vi "Unregister User Event.vi"(8 "error in (no error)":errorcluster, 10 "Event Registration in":refnum<event-registration>, 11 "Session in":refnum<k21>) -> (0 "error out":errorcluster, 3 "Session out":refnum<k21>)   [LabVIEW 2020, in "nisyscfg.lvlib"]
uses:
  <vilib>/nisyscfg/nisyscfg.lvlib
  <vilib>/nisyscfg/User Event.ctl
panel:
  in  "System Configuration":refnum<user-event>
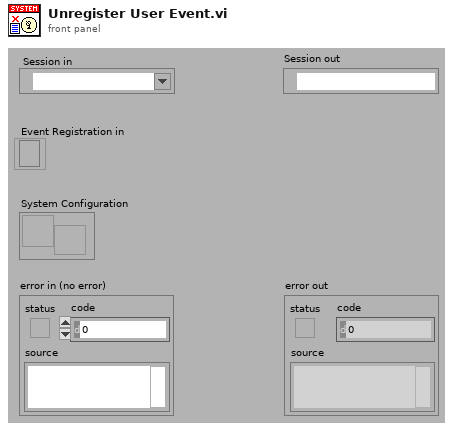
[diagram p1: front panel]
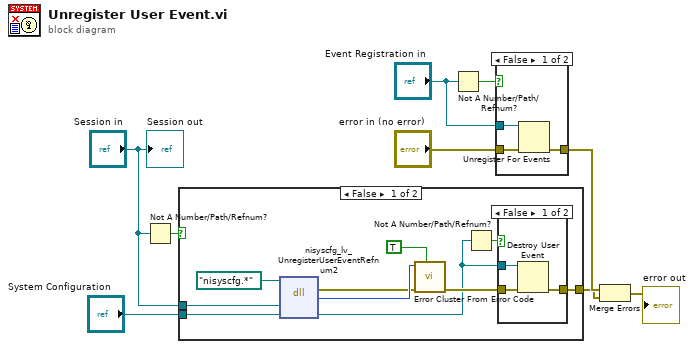
[diagram p0: block diagram]
diagram:
  n1 = Not A Number/Path/Refnum?(number/path/refnum="Session in") -> (NaN/Path/Refnum?=w5:bool)
  n2 = case shown="False" w5 {
    tunnel: [w13 _] -> w2
    tunnel: "Session in" -> [w17 _]
    tunnel: "System Configuration" -> [w12 _]
    frame False {
      n3 = dll-call lib="nisyscfg.*" fn="nisyscfg_lv_UnregisterUserEventRefnum2" label="Unregister User Event"(path in=path "nisyscfg.*", "system"=w17, "event"=w12) -> (error out=w18:errorcluster, "result"=w19:i32, "event"=w10:refnum<user-event>)  [unwired: 3 in, 1 out]
      n4 = call <vilib>:"Error Cluster From Error Code.vi"("show call chain? (False)"=TRUE, "error in (no error)"=w18, "error code (0)"=w19) -> ("error out"=w14:errorcluster)  [unwired: 6 in]
      n5 = Not A Number/Path/Refnum?(number/path/refnum=w10) -> (NaN/Path/Refnum?=w11:bool)
      n6 = case shown="False" w11 {
        tunnel: w14 -> [w22 w23]
        tunnel: [w21 w23] -> w13
        tunnel: w10 -> [w20 _]
        frame False {
          n7 = Destroy User Event(user event=w20, error in=w22) -> (error out=w21:errorcluster)
        }
        frame True {
        }
      }
    }
    frame True {
    }
  }
  n8 = Not A Number/Path/Refnum?(number/path/refnum="Event Registration in") -> (NaN/Path/Refnum?=w7:bool)
  n9 = case shown="False" w7 {
    tunnel: "error in (no error)" -> [w26 w27]
    tunnel: [w25 w27] -> w3
    tunnel: "Event Registration in" -> [w24 _]
    frame False {
      n10 = Unregister For Events(event registration refnum=w24, error in=w26) -> (error out=w25:errorcluster)
    }
    frame True {
    }
  }
  n11 = Merge Errors(w3, w2) -> (→"error out":errorcluster)
  "Session out" <- "Session in"
